vi "Dialog Tester - back to back.vi"() -> ()   [LabVIEW 2019]
doc: "<b>TEST VI</b> meant to see if data is properly cleared when popups are called in succession"
uses:
  Graphics.ctl
  Custom/Custom - Input (DBL)/Custom - Input (DBL).lvclass
  Custom/Custom - Input (I32)/Custom - Input (I32).lvclass
  Custom/Custom - Input (String)/Custom - Input (String).lvclass
  Custom/Custom - One Button/Custom - One Button.lvclass
  Custom/Custom - Timeout/Custom - Timeout.lvclass
  Custom/Custom - Timeout One Button/Custom - Timeout One Button.lvclass
  Custom/Custom - Timeout Two Button/Custom - Timeout Two Button.lvclass
  Custom/Custom - Two Button/Custom - Two Button.lvclass
  Standard/Timeout/Timeout.lvclass
  Pop-Up.lvlib
panel:
  in  "loop count":i32=8
  out "iteration":i32
  in  "Pop Up Type":enum16{"Custom", "Standard"}(ring)=enum."Standard"
  in  "Error In":errorcluster
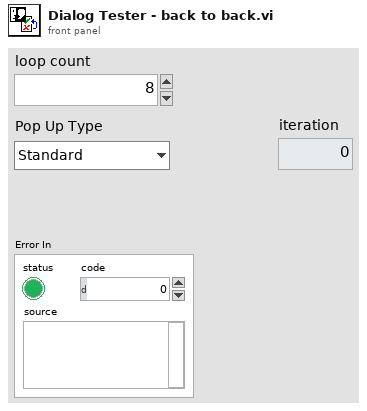
[diagram p1: front panel]
types:
  T1 = typedef "Pop-Up.lvlib/Graphics.ctl" = string
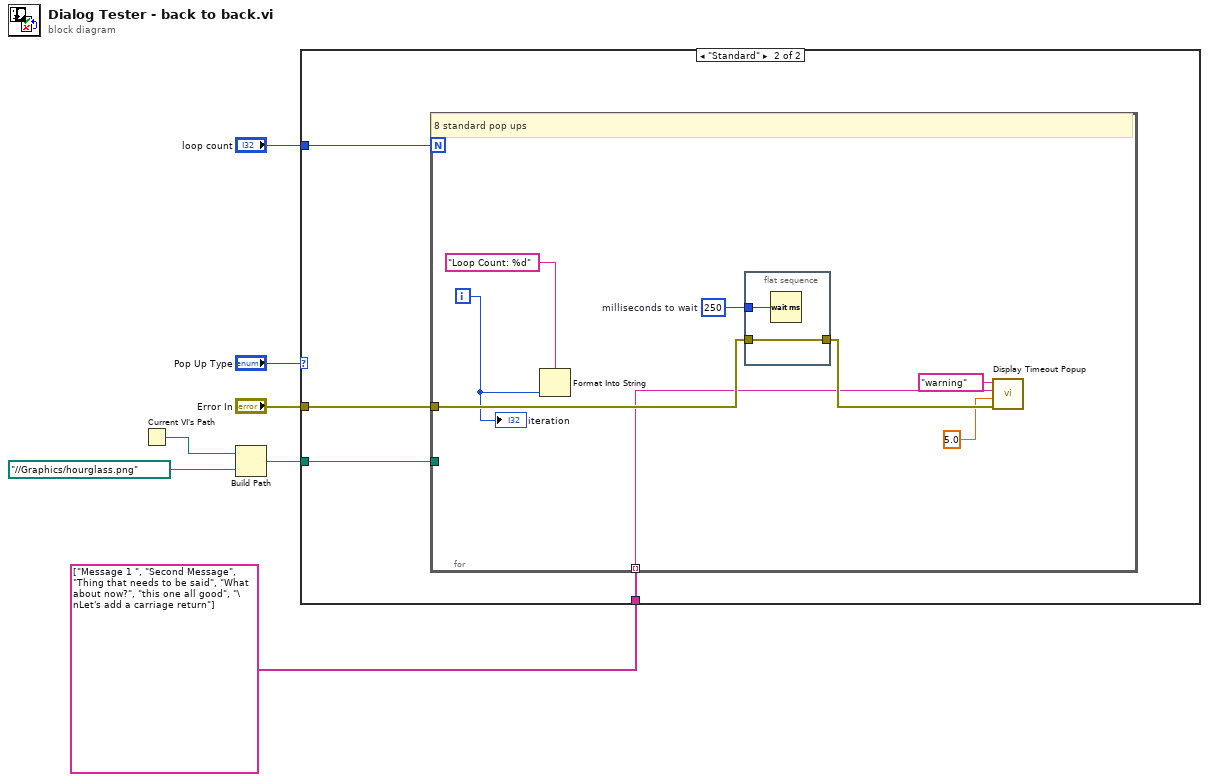
[diagram p0: block diagram]
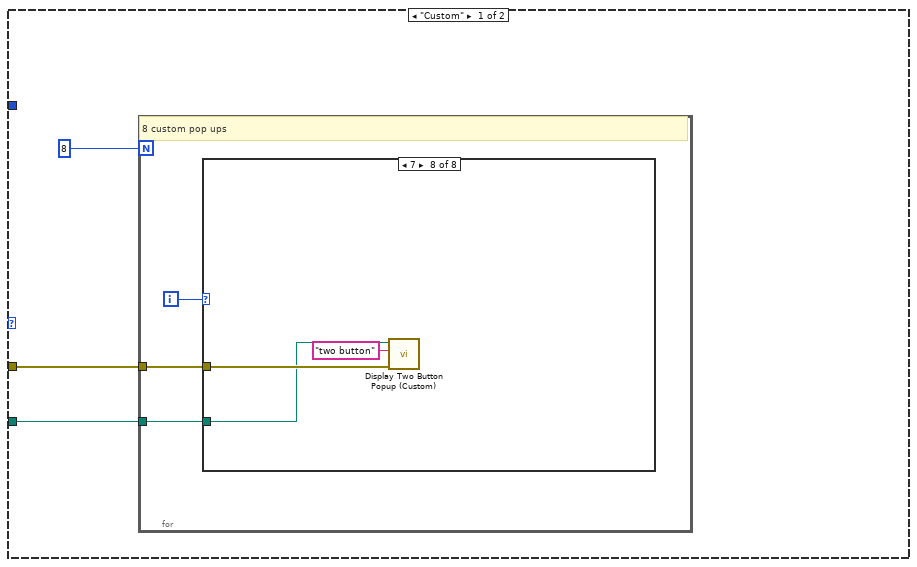
[diagram p2: hidden frame]
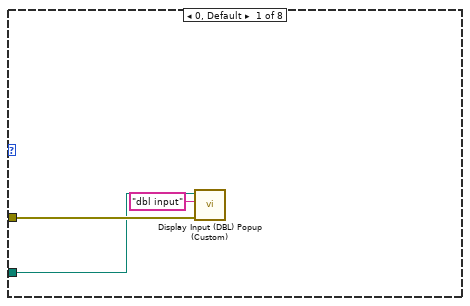
[diagram p3: hidden frame]
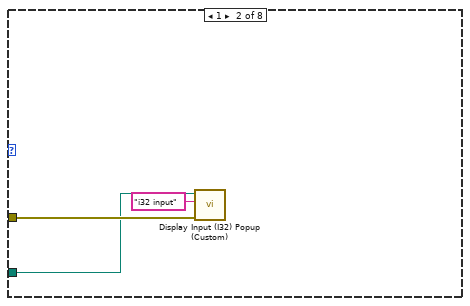
[diagram p4: hidden frame]
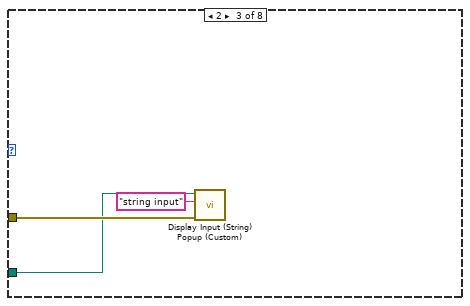
[diagram p5: hidden frame]
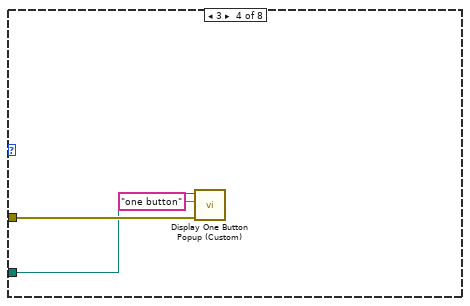
[diagram p6: hidden frame]
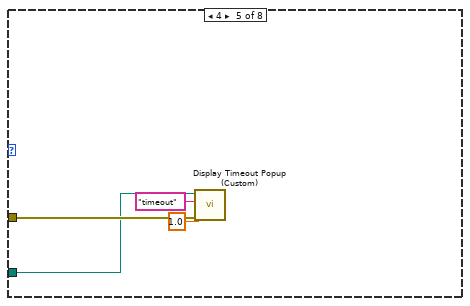
[diagram p7: hidden frame]
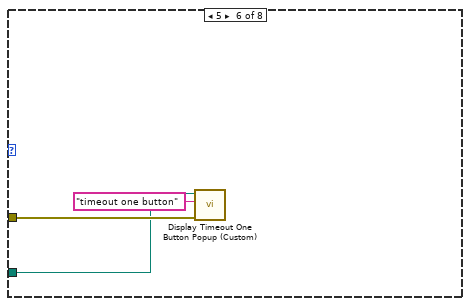
[diagram p8: hidden frame]
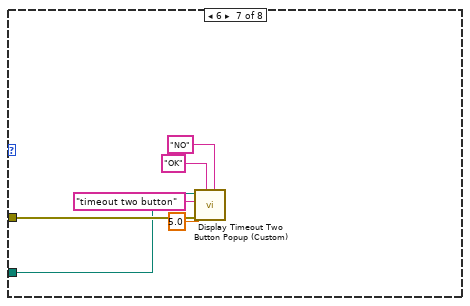
[diagram p9: hidden frame]
diagram:
  n1 = Current VI's Path() -> (path=w7:path)
  n2 = Build Path(base path=w7, name or relative path=path "../../Graphics/hourglass.png") -> (appended path=w5:path)
  n3 = case shown="\"Standard\"" "Pop Up Type" {
    tunnel: w5 -> [w9 w45]
    tunnel: "Error In" -> [w8 w44]
    tunnel: "loop count" -> [_ w43]
    tunnel: string[] ["Message 1 ", "Second Message", "Thing that needs to be said", "What about now?", "this one all good", "\nLet's add a carriage return"] -> [_ w42]
    frame "Custom" {
      n4 = for {
        N: 8 -> [_]
        tunnel: w9 -> [w12]
        tunnel: w8 -> [w11]
        i -> [w13]
        # "8 custom pop ups"
        n5 = case shown="7" w13 {
          tunnel: w12 -> [w15 w18 w21 w24 w28 w31 w37 w40]
          tunnel: w11 -> [w16 w19 w22 w25 w29 w32 w38 w41]
          frame 0, Default {
            n6 = call "Display Input (DBL) Popup (Custom).vi"("Error In"=w16, "Message"="dbl input", "Graphic"=w15) -> ()  [unwired: 7 in, 2 out]
          }
          frame 1 {
            n7 = call "Display Input (I32) Popup (Custom).vi"("Error In"=w19, "Message"="i32 input", "Graphic"=w18) -> ()  [unwired: 7 in, 2 out]
          }
          frame 2 {
            n8 = call "Display Input (String) Popup (Custom).vi"("Error In"=w22, "Message"="string input", "Graphic"=w21) -> ()  [unwired: 7 in, 2 out]
          }
          frame 3 {
            n9 = call "Display One Button Popup (Custom).vi"("Error In"=w25, "Message"="one button", "Graphic"=w24) -> ()  [unwired: 8 in, 1 out]
          }
          frame 4 {
            n10 = call "Display Timeout Popup (Custom).vi"("Error In"=w29, "Timeout (s)"=1.0, "Message"="timeout", "Graphic"=w28) -> ()  [unwired: 6 in, 2 out]
          }
          frame 5 {
            n11 = call "Display Timeout One Button Popup (Custom).vi"("Error In"=w32, "Message"="timeout one button", "Graphic"=w31) -> ()  [unwired: 7 in, 2 out]
          }
          frame 6 {
            n12 = call "Display Timeout Two Button Popup (Custom).vi"("N-Text"="NO", "Y-Text"="OK", "Error In"=w38, "Timeout (s)"=5.0, "Message"="timeout two button", "Graphic"=w37) -> ()  [unwired: 3 in, 3 out]
          }
          frame 7 {
            n13 = call "Display Two Button Popup (Custom).vi"("Error In"=w41, "Message"="two button", "Graphic"=w40) -> ()  [unwired: 7 in, 2 out]
          }
        }
      }
    }
    frame "Standard" {
      n14 = for {
        N: w43 -> [_]
        tunnel: w45 -> [_]
        tunnel: w44 -> [w53]
        tunnel: w42 -> [w48] mode=indexing
        i -> [w51]
        w50 = u32 250  # milliseconds to wait
        # "8 standard pop ups"
        n15 = Format Into String(format string="Loop Count: %d", w51) -> ()  [unwired: 2 in, 2 out]
        n16 = flat-sequence {
          tunnel: w50 -> [w55]
          tunnel: [w54] -> w49
          tunnel: w53 -> [w54]
          frame #0 {
            n17 = Wait (ms)(milliseconds to wait=w55) -> ()  [unwired: 1 out]
          }
        }
        n18 = call "Display Timeout Popup.vi"("error in"=w49, "Timeout (s)"=5.0, "Message"=w48, "Graphic"=T1 "warning") -> ()  [unwired: 6 in, 2 out]
        "iteration" <- w51
      }
    }
  }
